vi "4155C Config Display add.vi"(4 "Ymax":dbl format="%.2e", 6 "Ymin":dbl format="%.2e", 7 "SMU4":bool, 8 "error in (no error)":errorcluster, 9 "Logarithmic":bool=TRUE, 10 "SPA Display":bool, 11 "VISA session":refnum<visa-resource-name>) -> (0 "error out":errorcluster, 3 "dup VISA resource name":refnum<visa-resource-name>)   [LabVIEW 2019]
doc: "This VI configures the timing parameters of the measurement functions. The settings of this VI could be different from the actual instrument's settings due to limits imposed by other parameters inside the instrument. To check the actual values of integration time and number of power line cycles, run HP415xA Query Integration Time.vi."
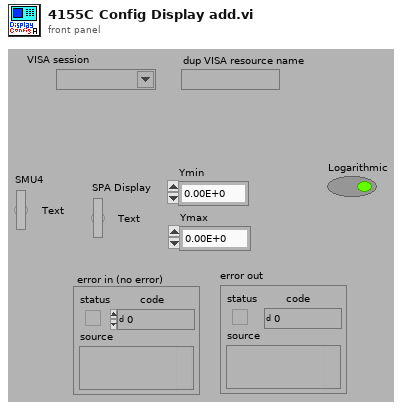
[diagram p1: front panel]
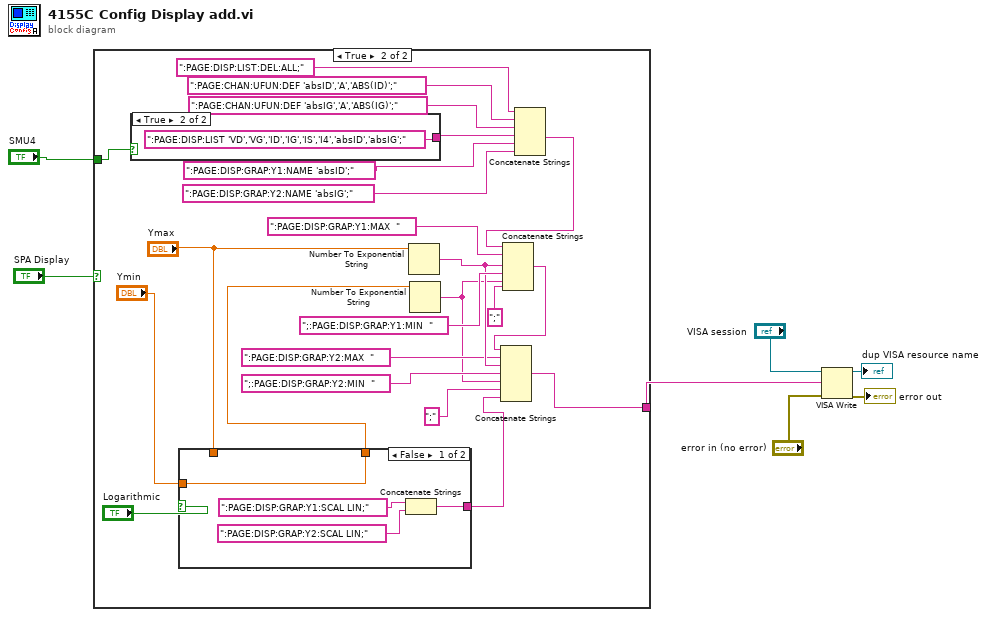
[diagram p0: block diagram]
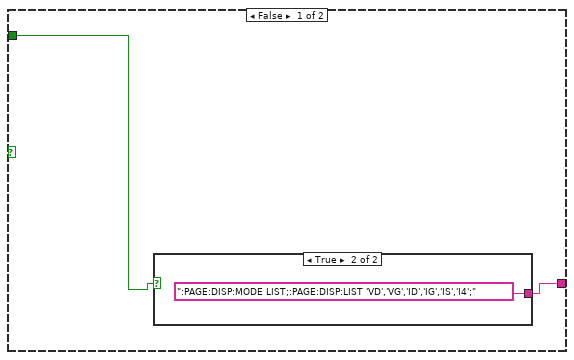
[diagram p2: hidden frame]
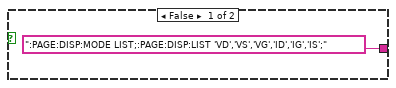
[diagram p3: hidden frame]
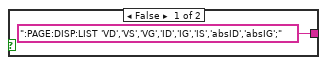
[diagram p4: hidden frame]
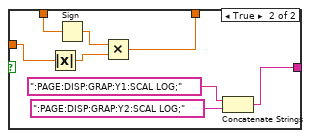
[diagram p5: hidden frame]
diagram:
  n1 = case shown="True" "SPA Display" {
    tunnel: [w9 w21] -> w5
    tunnel: "SMU4" -> [w8 w13]
    frame False {
      n2 = case shown="True" w8 {
        tunnel: [":PAGE:DISP:MODE LIST;:PAGE:DISP:LIST 'VD','VS','VG','ID','IG','IS';" ":PAGE:DISP:MODE LIST;:PAGE:DISP:LIST 'VD','VG','ID','IG','IS','I4';"] -> w9
        frame False {
        }
        frame True {
        }
      }
    }
    frame True {
      n3 = case shown="True" w13 {
        tunnel: [":PAGE:DISP:LIST 'VD','VS','VG','ID','IG','IS','absID','absIG';" ("write buffer (\"\")") ":PAGE:DISP:LIST 'VD','VG','ID','IG','IS','I4','absID','absIG';" ("write buffer (\"\")")] -> w14
        frame False {
        }
        frame True {
        }
      }
      n4 = case shown="False" "Logarithmic" {
        tunnel: [w39 w41] -> w20
        tunnel: "Ymax" -> [_ w46]
        tunnel: "Ymin" -> [w40 w45]
        tunnel: [w40 w44] -> w26
        frame False {
          n5 = Concatenate Strings(":PAGE:DISP:GRAP:Y1:SCAL LIN;", ":PAGE:DISP:GRAP:Y2:SCAL LIN;") -> (w39:string)
        }
        frame True {
          n6 = Absolute Value(x=w45) -> (abs(x)=w48:dbl)
          n7 = Sign(1:w46) -> (0:w47:dbl)
          n8 = Multiply(x=w47, y=w48) -> (x*y=w44:dbl)
          n9 = Concatenate Strings(":PAGE:DISP:GRAP:Y1:SCAL LOG;", ":PAGE:DISP:GRAP:Y2:SCAL LOG;") -> (w41:string)
        }
      }
      n10 = Number To Exponential String(number="Ymax") -> (E-format string=w19:string)  [unwired: 3 in]
      n11 = Number To Exponential String(number=w26) -> (E-format string=w15:string)  [unwired: 3 in]
      n12 = Concatenate Strings(":PAGE:DISP:LIST:DEL:ALL;" ("write buffer (\"\")"), ":PAGE:CHAN:UFUN:DEF 'absID','A','ABS(ID)';" ("write buffer (\"\")"), ":PAGE:CHAN:UFUN:DEF 'absIG','A','ABS(IG)';" ("write buffer (\"\")"), w14, ":PAGE:DISP:GRAP:Y1:NAME 'absID';" ("write buffer (\"\")"), ":PAGE:DISP:GRAP:Y2:NAME 'absIG';" ("write buffer (\"\")")) -> (w30:string)
      n13 = Concatenate Strings(w30, ":PAGE:DISP:GRAP:Y1:MAX  " ("write buffer (\"\")"), w19, ";:PAGE:DISP:GRAP:Y1:MIN  " ("write buffer (\"\")"), w15, ";" ("Substring")) -> (w22:string)
      n14 = Concatenate Strings(w22, ":PAGE:DISP:GRAP:Y2:MAX  " ("write buffer (\"\")"), w19, ";:PAGE:DISP:GRAP:Y2:MIN  " ("write buffer (\"\")"), w15, ";" ("Substring"), w20) -> (w21:string)
    }
  }
  n15 = VISA Write(VISA resource name="VISA session", write buffer=w5, error in (no error)="error in (no error)") -> (VISA resource name out=→"dup VISA resource name":refnum<visa-resource-name>, error out=→"error out":errorcluster)  [unwired: 1 out]
